vi "Passing Paramters String.vi"(11 "str":string) -> (2 "function return":i32, 3 "str out":string)   [LabVIEW 2018, in "ParsingDataSampleDLL.lvlib"]
doc: "__declspec(dllexport) int PassingParamters_String (char *str);"
uses:
  ParsingDataSampleDLL.lvlib
  ni_reference_vs/Debug/ParsingDataSampleDLL.dll
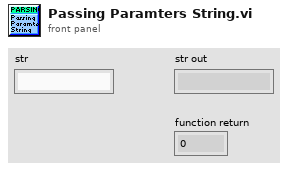
[diagram p1: front panel]
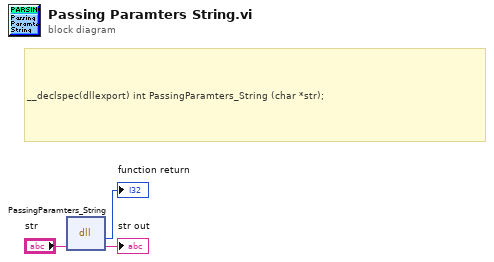
[diagram p0: block diagram]
diagram:
  # "__declspec(dllexport) int PassingParamters_String (char *str);"
  n1 = dll-call lib="C:/Users/celit/Documents/GitHub/Labview_Python_DLL_Call/ni_reference_vs/Debug/ParsingDataSampleDLL.*" fn="PassingParamters_String"("str"="str") -> (→"function return":i32, "str"=→"str out":string)  [unwired: 3 in, 2 out]
